vi "NIMS_Check DAQ.vi"() -> (3 "DAQ present?":bool)   [LabVIEW 2021]
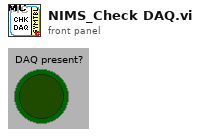
[diagram p1: front panel]
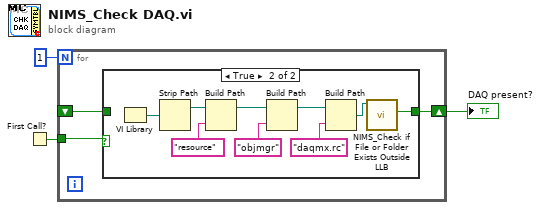
[diagram p0: block diagram]
diagram:
  n1 = First Call?() -> (First Call?: T/F=w3:bool)
  n2 = for {
    N: 1 -> [_]
    tunnel: w3 -> [w6]
    shift-right: [w5] -> w1
    shift-left: _ -> [w4]
    n3 = case shown="True" w6 {
      tunnel: [w7 w9] -> w5
      tunnel: w4 -> [w7 _]
      frame False {
      }
      frame True {
        n4 = VI Library() -> (path=w16:path)
        n5 = Strip Path(path=w16) -> (stripped path=w15:path)  [unwired: 1 out]
        n6 = Build Path(base path=w15, name or relative path="resource") -> (appended path=w13:path)
        n7 = Build Path(base path=w13, name or relative path="objmgr") -> (appended path=w11:path)
        n8 = Build Path(base path=w11, name or relative path="daqmx.rc") -> (appended path=w8:path)
        n9 = call <vilib>:"NIMS_Check if File or Folder Exists Outside LLB.vi"("path"=w8) -> ("file or folder exists?"=w9:bool)  [unwired: 8 in, 2 out]
      }
    }
  }
  "DAQ present?" <- w1
